vi "DataLengthBytes.vi"(11 "Data":string) -> (3 "Length Bytes":string)   [LabVIEW 2013, in "WebSockets.lvlib"]
doc: "Generates the message length bytes of the WebSockets packet. A varying number of bytes is used to indicate the length of the data."
uses:
  WebSockets.lvlib
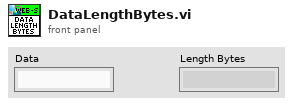
[diagram p1: front panel]
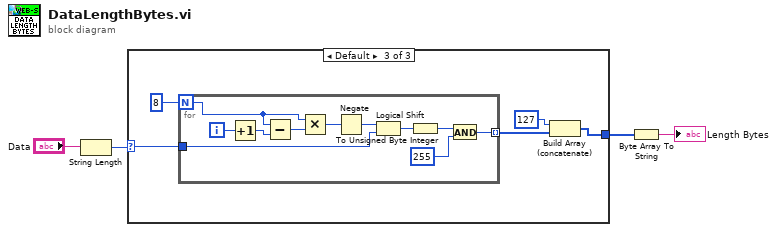
[diagram p0: block diagram]
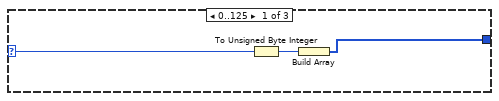
[diagram p2: hidden frame]
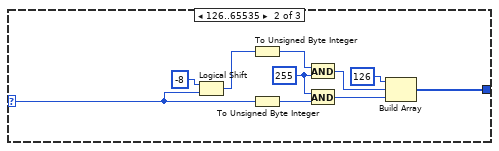
[diagram p3: hidden frame]
diagram:
  n1 = String Length(string="Data") -> (length=w4:i32)
  n2 = case shown="Default" w4 {
    selector: w4 -> [w7 w8 w18]
    tunnel: [w5 w17 w21] -> w2
    frame 0..125 {
      n3 = To Unsigned Byte Integer(number=w7) -> (unsigned 8bit integer=w6:u8)
      n4 = Build Array(w6) -> (w5:u8[])
    }
    frame 126..65535 {
      w10 = u8 255 ("y")
      n5 = Logical Shift(y=i16 -8, x=w8) -> (x << y=w14:i32)
      n6 = To Unsigned Byte Integer(number=w14) -> (unsigned 8bit integer=w13:u8)
      n7 = To Unsigned Byte Integer(number=w8) -> (unsigned 8bit integer=w9:u8)
      n8 = And(x=w13, y=w10) -> (x .and. y?=w12:u8)
      n9 = And(x=w10, y=w9) -> (x .and. y?=w11:u8)
      n10 = Build Array(u8 126, w12, w11) -> (w17:u8[])
    }
    frame Default {
      n11 = for {
        N: 8 -> [w25]
        tunnel: [w30] -> w19 mode=indexing
        tunnel: w18 -> [w33]
        i -> [w28]
        n12 = Increment(x=w28) -> (x+1=w27:i32)
        n13 = Subtract(x=w25, y=w27) -> (x-y=w26:i32)
        n14 = Multiply(x=w25, y=w26) -> (x*y=w24:i32)
        n15 = Negate(x=w24) -> (-x=w23:i32)
        n16 = Logical Shift(y=w23, x=w33) -> (x << y=w32:i32)
        n17 = To Unsigned Byte Integer(number=w32) -> (unsigned 8bit integer=w31:u8)
        n18 = And(x=w31, y=u8 255) -> (x .and. y?=w30:u8)
      }
      n19 = Build Array (concatenate)(u8 127, w19) -> (w21:u8[])
    }
  }
  n20 = Byte Array To String(unsigned byte array=w2) -> (string=→"Length Bytes":string)
